vi "Expansion Enqueue.vi"(7 "Opposite End? (F)":bool, 8 "error in (no error)":errorcluster, 9 "Variant":variant, 10 "State":T1, 11 "Queue in":refnum<queue>) -> (0 "error out":errorcluster, 3 "Queue out":refnum<queue>)   [LabVIEW 2017, in "Expansion.lvclass"]
uses:
  Expansion.lvclass
  Type Defs/Expansion State.ctl
  Expansion.lvclass/Expansion.ctl
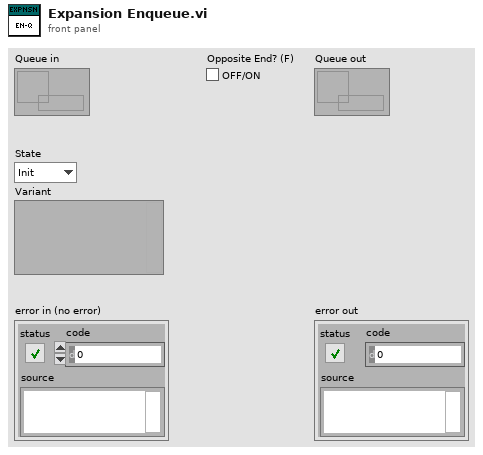
[diagram p1: front panel]
types:
  T1 = typedef "Expansion.lvclass/Expansion State.ctl" = enum16{"Init", "Update", "Go", "Move from Load to Heating", "Stop Motor", "Operate Cylinders", "Wait and Monitor", "Move from Heating to Unload", "Unload", "Move from Unload to Heating", "Move from Heating to Load", "Complete Process", "Stop", "Idle", "Error", "Shutdown"}
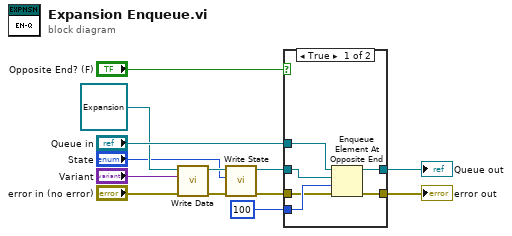
[diagram p0: block diagram]
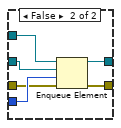
[diagram p2: hidden frame]
diagram:
  n1 = call "Write Data.vi"("error in (no error)"="error in (no error)", "Data"="Variant", "Expansion in"=refnum<class "Expansion.lvclass"> refnum) -> ("error out"=w7:errorcluster, "Expansion out"=w10:refnum<class "Expansion.lvclass">)  [unwired: 7 in]
  n2 = call "Write State.vi"("error in (no error)"=w7, "State"="State", "Expansion in"=w10) -> ("error out"=w8:errorcluster, "Expansion out"=w9:refnum<class "Expansion.lvclass">)  [unwired: 7 in]
  n3 = case shown="True" "Opposite End? (F)" {
    tunnel: [w19 w25] -> w13
    tunnel: "Queue in" -> [w18 w24]
    tunnel: 100 ("timeout in ms (-1)") -> [w17 w23]
    tunnel: w9 -> [w16 w22]
    tunnel: w8 -> [w15 w21]
    tunnel: [w14 w20] -> w4
    frame True {
      n4 = Enqueue Element At Opposite End(queue=w18, element=w16, timeout in ms (-1)=w17, error in (no error)=w15) -> (queue out=w19:refnum<queue>, error out=w14:errorcluster)  [unwired: 1 out]
    }
    frame False {
      n5 = Enqueue Element(queue=w24, element=w22, timeout in ms (-1)=w23, error in (no error)=w21) -> (queue out=w25:refnum<queue>, error out=w20:errorcluster)  [unwired: 1 out]
    }
  }
  "error out" <- w4
  "Queue out" <- w13
